vi "computeLCs.vi"(8 "error in (no error)":errorcluster, 11 "LaguerreDeconClass in":refnum<class "LaguerreDeconEngineClass.lvclass">) -> (0 "error out":errorcluster, 3 "LaguerreDeconClass out":refnum<class "LaguerreDeconEngineClass.lvclass">)   [LabVIEW 2020, in "LaguerreDeconEngineClass.lvclass"]
uses:
  LaguerreDeconEngineClass.lvclass
  LaguerreDeconEngineClass.lvclass/LaguerreDeconEngineClass.ctl
  LaguerreDeconLib.lvlib
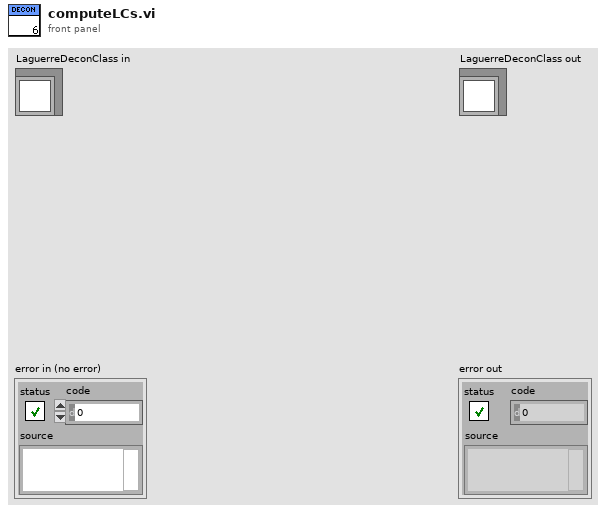
[diagram p1: front panel]
types:
  T1 = cluster{"LGBasisRows":u64, "LGBasisCols":u64, "vvRows":u64, "vvCols":u64, "DRows":u64, "DCols":u64, "LHS_Multi_Rows":u64, "LHS_Multi_Cols":u64, "RHS_Multi_Rows":u64, "RHS_Multi_Cols":u64, "lam length":u64, "LCs length":u64}
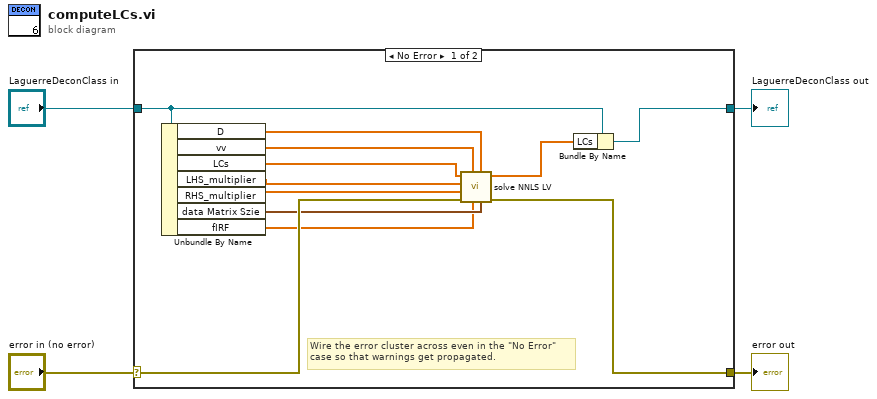
[diagram p0: block diagram]
diagram:
  n1 = case shown="No Error" "error in (no error)" {
    selector: "error in (no error)" -> [w13 w18]
    tunnel: [w12 w18] -> w3
    tunnel: [w8 w17] -> w1
    tunnel: "LaguerreDeconClass in" -> [w7 w17]
    frame No Error {
      # "Wire the error cluster across even in the \"No Error\"\ncase so that warnings get propagated."
      n2 = Unbundle By Name(w7) -> ("D"=w10:dbl[], "vv"=w11:dbl[], "LCs"=w16:dbl[], "LHS_multiplier"=w15:dbl[], "RHS_multiplier"=w14:dbl[], "data Matrix Szie"=w9:T1, "fIRF"=w5:dbl[])
      n3 = call "solve NNLS LV.vi"("data Matrix Szie"=w9, "D"=w10, "fIRF"=w5, "vv"=w11, "error in (no error)"=w13, "RHS_multiplier_array"=w14, "LHS_multiplier_array"=w15, "LCs"=w16) -> ("error out"=w12:errorcluster, "LCs out"=w6:dbl[])  [unwired: 2 out]
      n4 = Bundle By Name(cluster=w7, "LCs"=w6) -> (w8:refnum<class "LaguerreDeconEngineClass.lvclass">)
    }
    frame Error {
    }
  }
  "error out" <- w3
  "LaguerreDeconClass out" <- w1
